vi "Parse updateDeleteMessages.vi"(8 "error in (no error)":errorcluster, 11 "JSON (UTF-8) String":string) -> (0 "error out":errorcluster, 2 "Telegram State":T1, 3 "Variant":variant)   [LabVIEW 2015, in "JSON Library.lvlib"]
doc: "Created IvanLis by LabVIEW Portal\nProfile: http://labviewportal.org/memberlist.php?mode=viewprofile&u=987\neMail: IvanLisanov@gMail.com\nTelegram: https://t.me/IvanLis"
uses:
  JSON Library.lvlib
  Telegram Library/TypeDef/Telegram State.ctl
  TypeDef/Delete Messages.ctl
  Telegram Library/Telegram Library.lvlib
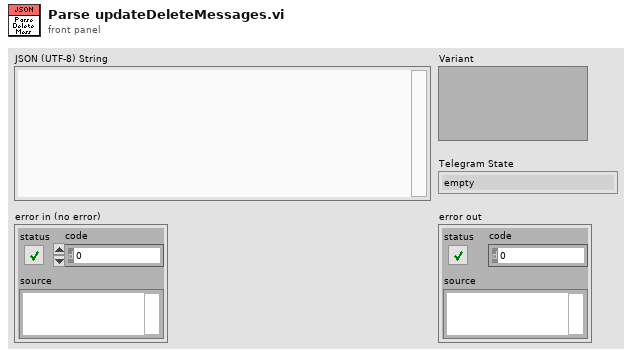
[diagram p1: front panel]
types:
  T1 = typedef "Telegram Library.lvlib/Telegram State.ctl" = enum16{"empty", "ok", "authorizationStateClosed", "authorizationStateWaitTdlibParameters", "authorizationStateWaitEncryptionKey", "authorizationStateWaitPhoneNumber", "authorizationStateWaitCode", "connectionStateWaitingForNetwork", "connectionStateConnectingToProxy", "connectionStateUpdating", "connectionStateConnecting", "connectionStateReady", "updateUser_user", "updateNewChat_chat", "updateNewMessage_Text", "updateChatLastMessage_Text", "updateDeleteMessages", "updateChatPosition", "ChatHistoryMessages_Text"}
  T2 = typedef "JSON Library.lvlib/Delete Messages.ctl" = cluster{"@type":string, "chat_id":i64, "message_ids":i64[]}
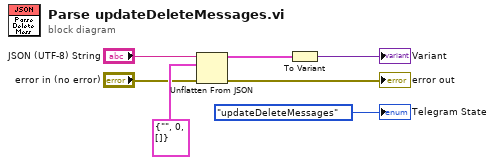
[diagram p0: block diagram]
diagram:
  n1 = Unflatten From JSON(JSON string="JSON (UTF-8) String", type and defaults=T2 {"@type"="", "chat_id"=0, "message_ids"=[]} ("Message"), error in (no error)="error in (no error)") -> (value=w6:T2, error out=→"error out":errorcluster)  [unwired: 4 in]
  n2 = To Variant(anything=w6) -> (Variant=→"Variant":variant)
  "Telegram State" <- Telegram_State."updateDeleteMessages" ("Telegram State")
